vi "Tree Data Lookup.vi"(11 "Tag in":string) -> (0 "Found?":bool, 1 "Tree Index Enum":T1=enum."Analog Values", 2 "Tag out":string, 3 "Tree Data":T2 {"Data Type" items=["Tree Parent"=-1, "Numeric"=0, "String"=1, "Boolean"=2, "Enum"=3]}, 4 "Item Number":i32, 5 "Tree Label":string)   [LabVIEW 2020, in "Output Sequencer.lvlib" / "Settings UI.lvclass"]
uses:
  Settings UI.lvclass
  Types/Tree Item Settings.ctl
  Types/Data Type.ctl
  Types/Tree Index Enum.ctl
  Globals/Global Tree Data.vi
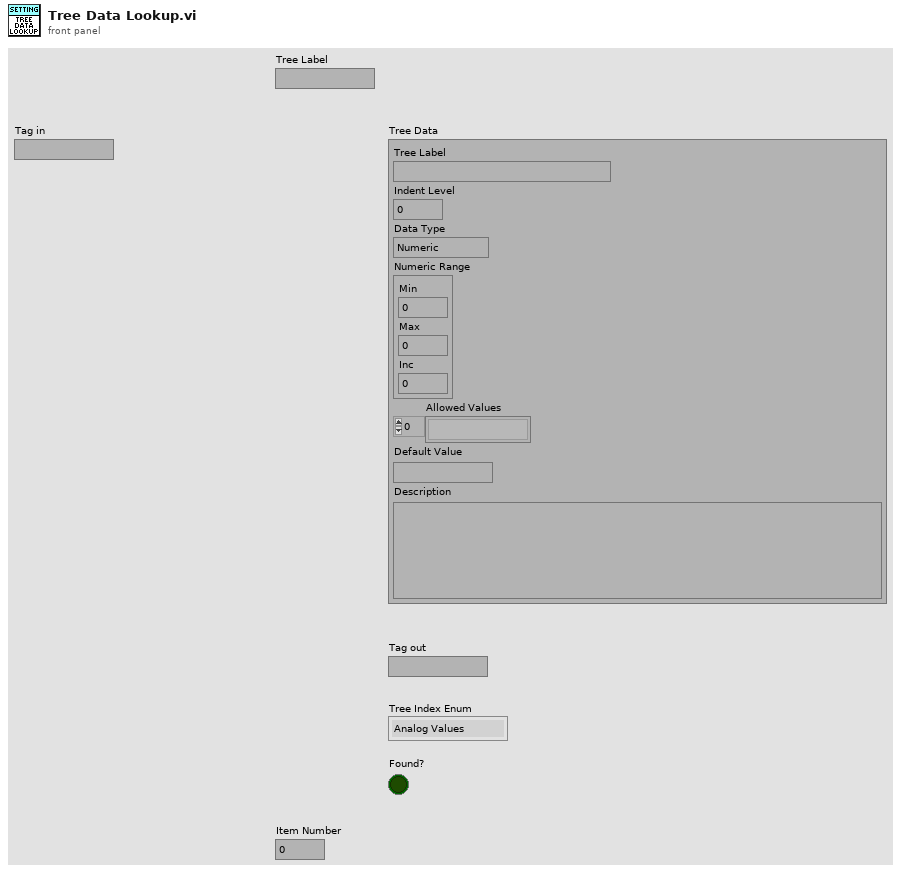
[diagram p1: front panel]
types:
  T1 = typedef "Output Sequencer.lvlib/Settings UI.lvclass/Tree Index Enum.ctl" = enum16{"General Settings", "Num Steps", "Num Analog", "Num Digital", "Show Confirmation", "Interp Priority", "Adv Timing", "Enable Conditions", "Seq Execution", "Reset Test Start", "Only When Test", "Delay After Test", "Start condition", "Re-triggering", "Stop condition", "Stop After Cycles", "Stop Values", "Default Values", "Default Analog", "Default Digital", "Steps", "Step #", "Description", "Precondition", "Duration", "Mode", "Delay Between Vals", "Analog Values", "Digital Values", "Postcondition", "On True", "On False"}
  T2 = typedef "Output Sequencer.lvlib/Settings UI.lvclass/Tree Item Settings.ctl" = cluster{"Tree Label":string, "Indent Level":i32, "Data Type":T3, "Numeric Range":cluster{"Min":dbl, "Max":dbl, "Inc":dbl}, "Allowed Values":string[], "Default Value":string, "Description":string}
  T3 = typedef "Output Sequencer.lvlib/Settings UI.lvclass/Data Type.ctl" = i16
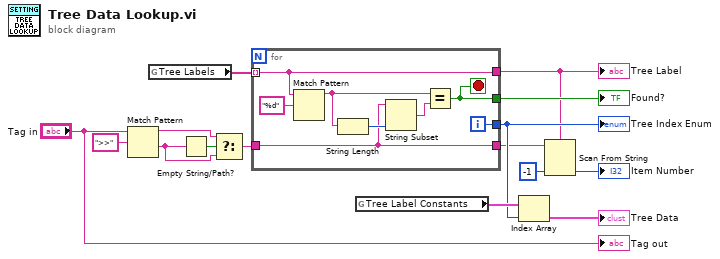
[diagram p0: block diagram]
diagram:
  n1 = Match Pattern(string="Tag in", regular expression=">>") -> (before substring=w11:string, after substring=w9:string)  [unwired: 1 in, 2 out]
  n2 = global read "Global Tree Data.vi" "Tree Labels"() -> (w13:string[])
  n3 = Empty String/Path?(string/path=w9) -> (empty?=w10:bool)
  n4 = Select(t=w11, s=w10, f=w9) -> (s? t:f=w8:string)
  n5 = for {
    tunnel: w13 -> [w17] mode=indexing
    tunnel: w8 -> [w16]
    tunnel: [w20] -> w7
    tunnel: [w17] -> w5
    tunnel: [w18] -> w6
    tunnel: [w16] -> w4
    i -> [w20]
    stop <- w18 stop-if-true
    n6 = Match Pattern(string=w17, regular expression="%d") -> (before substring=w19:string)  [unwired: 1 in, 3 out]
    n7 = String Length(string=w19) -> (length=w22:i32)
    n8 = String Subset(string=w16, length (rest)=w22) -> (substring=w21:string)  [unwired: 1 in]
    n9 = Equal?(x=w19, y=w21) -> (x = y?=w18:bool)
  }
  "Tree Label" <- w5
  "Tree Index Enum" <- w7
  "Found?" <- w6
  n10 = global read "Global Tree Data.vi" "Tree Label Constants"() -> (w14:T2[])
  n11 = Index Array(array=w14, index=w7) -> (element=→"Tree Data":T2)
  n12 = Scan From String(format string=w5, input string=w4, default 1=-1 ("default (0 I32)")) -> (output 1=→"Item Number":i32)  [unwired: 2 in, 3 out]
  "Tag out" <- "Tag in"
